vi "I2C Close.vi"(7 "I2C Channel (0)":u8, 8 "Error In":errorcluster, 11 "LINX Resource":T1) -> (0 "Error Out":errorcluster, 3 "LINX Resource":T1)   [LabVIEW 2013, in "LVH-LINX.lvlib"]
doc: "Close the specified I2C channel."
uses:
  LVH-LINX.lvlib
  Private/Type Defs/LINX Ref.ctl
  Private/Type Defs/Platform.ctl
  Private/Type Defs/Interface.ctl
  Private/Device/Type Defs/LINX Device Config.ctl
  Private/Device/Type Defs/TCP Config.ctl
  Private/Type Defs/Device Family.ctl
  Private/Device/Type Defs/Channels.ctl
  Private/Type Defs/Peripheral.ctl
  Private/Type Defs/Channel FGV States.ctl
  <vilib>/myRIO/Instrument Drivers/Onboard IO/I2C/typedefs/I2C Transfer Rate.ctl
  <vilib>/myRIO/Instrument Drivers/Onboard IO/I2C/typedefs/I2C Configuration.ctl
  <vilib>/myRIO/Common/Instrument Driver Framework/myRIO v1.0/I2C/typedefs/I2C Channels Enum.ctl
  <vilib>/myRIO/Common/Instrument Driver Framework/Utilities/typedefs/Generic FPGA Reference.ctl
  <vilib>/myRIO/Common/Instrument Driver Framework/Utilities/typedefs/myRIO v1.0 Reference.ctl
  <vilib>/myRIO/Common/Instrument Driver Framework/Utilities/typedefs/Hardware Version Enum.ctl
  <vilib>/myRIO/Common/Instrument Driver Framework/Utilities/typedefs/myRIO Generic Hardware Reference.ctl
  <vilib>/myRIO/Instrument Drivers/Onboard IO/I2C/typedefs/I2C Reference.ctl
  Private/Device/Device.lvlib
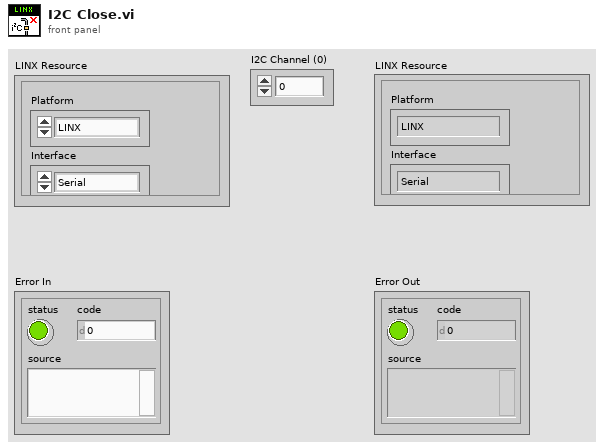
[diagram p1: front panel]
types:
  T1 = typedef "LVH-LINX.lvlib/LINX Ref.ctl" = cluster{"Platform":T2, "Interface":T3, "LINX Device Config":T4}
  T2 = typedef "LVH-LINX.lvlib/Platform.ctl" = enum16{"LINX", "myRIO"}
  T3 = typedef "LVH-LINX.lvlib/Interface.ctl" = enum16{"Serial", "TCP"}
  T4 = typedef "LVH-LINX.lvlib/Device.lvlib/LINX Device Config.ctl" = cluster{"Interface":T3, "COM Port":refnum<visa-resource-name>, "TCP Configuration":T5, "Device Family":T6, "Device ID":u8, "Device Name":string, "TCP Ref":refnum<k5>, "Channels":T7}
  T5 = typedef "LVH-LINX.lvlib/Device.lvlib/TCP Config.ctl" = cluster{"IP Address":string, "Port":u16}
  T6 = typedef "LVH-LINX.lvlib/Device Family.ctl" = enum8{"National Instruments", "Digilent", "Arduino"}
  T7 = typedef "LVH-LINX.lvlib/Channels.ctl" = cluster{"DI Channels":u8[], "DO Channels":u8[], "AI":u8[], "AO":u8[], "PWM":u8[], "QE":u8[], "UART":u8[], "I2C 2":u8[], "SPI":u8[], "CAN":u8[], "AI Ref (V)":dbl, "AO Resolution (Bits)":u8, "AO Ref (V)":dbl}
  T8 = typedef "LVH-LINX.lvlib/Peripheral.ctl" = enum8{"DI", "DO", "AI", "AO", "PWM", "QE", "UART", "I2C", "SPI", "CAN"}
  T9 = typedef "LVH-LINX.lvlib/Channel FGV States.ctl" = enum16{"Initialize", "Get", "Set"}
  T10 = typedef "I2C.lvlib/I2C Reference.ctl" = cluster{"myRIO Reference":T11, "I2C Channels Enum":T15, "I2C Configuration":T16}
  T11 = typedef "myRIO Generic Hardware Reference.ctl" = cluster{"myRIO Model":T12, "myRIO Hardware Reference":T13}
  T12 = typedef "Hardware Version Enum.ctl" = enum16{"Unknown", "myRIO-1900", "myRIO-1950"}
  T13 = typedef "myRIO v1.0 Reference.ctl" = cluster{"Generic FPGA Reference":T14, "Allow multiple opens":bool}
  T14 = typedef "Generic FPGA Reference.ctl" = refnum<k20>
  T15 = typedef "I2C Channels Enum.ctl" = enum16{"Not Connected", "A/I2C", "B/I2C"}
  T16 = typedef "I2C.lvlib/I2C Configuration.ctl" = cluster{"I2C Transfer Rate":T17}
  T17 = typedef "I2C.lvlib/I2C Transfer Rate.ctl" = enum16{"Standard Mode (100 kbps)", "Fast Mode (400 kbps)"}
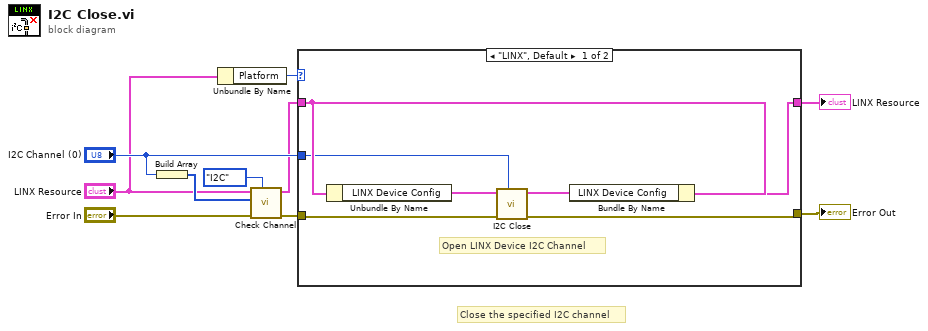
[diagram p0: block diagram]
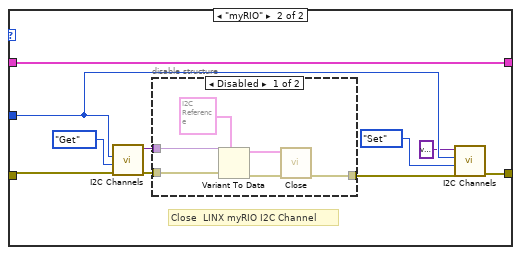
[diagram p2: hidden frame]
diagram:
  # "Close the specified I2C channel"
  n1 = Build Array("I2C Channel (0)") -> (w7:u8[])
  n2 = Unbundle By Name("LINX Resource") -> ("Platform"=w10:T2)
  n3 = call "Check Channel.vi"("Peripheral"=Peripheral."I2C", "Error In"="Error In", "Channels"=w7, "LINX Resource"="LINX Resource") -> ("Error Out"=w4:errorcluster, "LINX Resource"=w1:T1)  [unwired: 5 in, 1 out]
  n4 = case shown="\"LINX\", Default" w10 {
    tunnel: w4 -> [w12 w23]
    tunnel: w1 -> [w17 w27]
    tunnel: [w11 w26] -> w9
    tunnel: [w16 w27] -> w8
    tunnel: "I2C Channel (0)" -> [w13 w22]
    frame "LINX", Default {
      # "Open LINX Device I2C Channel"
      n5 = Unbundle By Name(w17) -> ("LINX Device Config"=w15:T4)
      n6 = call "I2C Close.vi"("I2C Channel"=w13, "Error In"=w12, "LINX Device Config"=w15) -> ("Error Out"=w11:errorcluster, "LINX Device Config"=w14:T4)  [unwired: 7 in]
      n7 = Bundle By Name(cluster=w17, "LINX Device Config"=w14) -> (w16:T1)
    }
    frame "myRIO" {
      # "Close  LINX myRIO I2C Channel"
      n8 = call "I2C Channels.vi"("Error In"=w23, "Channel State"=Channel_FGV_States."Get", "Channel Number"=w22) -> ("Error Out"=w20:errorcluster, "I2C Channel"=w21:variant)  [unwired: 7 in]
      n9 = disable-structure shown="Disabled" {
        disable-tunnel: w21 -> [w30 _]
        disable-tunnel: w20 -> [w29 _]
        disable-tunnel: [w28 _] -> w19
        frame Disabled {
          n10 = Variant To Data(error in=w29, type=T10 {"myRIO Reference"={"myRIO Model"=enum."Unknown", "myRIO Hardware Reference"={"Generic FPGA Reference"=refnum, "Allow multiple opens"=FALSE}}, "I2C Channels Enum"=enum."Not Connected", "I2C Configuration"={"I2C Transfer Rate"=enum."Standard Mode (100 kbps)"}}, Variant=w30) -> (data=w32:T10, error out=w31:errorcluster)
          n11 = call <vilib>:"Close.vi"("error in (no error)"=w31, "I2C Ref In"=w32) -> ("error out"=w28:errorcluster)  [unwired: 9 in]
        }
        frame Enabled {
        }
      }
      n12 = call "I2C Channels.vi"("Error In"=w19, "Channel State"=Channel_FGV_States."Set", "Channel Number"=w22, "I2C Channel"=variant) -> ("Error Out"=w26:errorcluster)  [unwired: 6 in, 1 out]
    }
  }
  "Error Out" <- w9
  "LINX Resource" <- w8
